vi "Get First Pt.vi"(11 "Input Traj":T1) -> (3 "First Traj Pt":dbl[](array[numeric]))   [LabVIEW 2016]
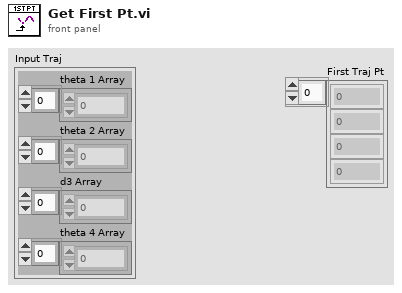
[diagram p1: front panel]
types:
  T1 = cluster{"theta 1 Array":dbl[], "theta 2 Array":dbl[], "d3 Array":dbl[], "theta 4 Array":dbl[]}
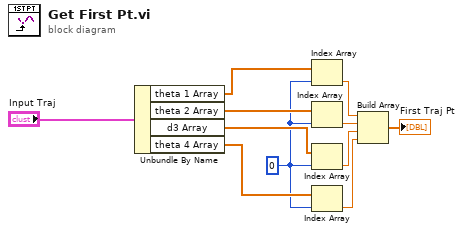
[diagram p0: block diagram]
diagram:
  w2 = 0 ("index")
  n1 = Unbundle By Name("Input Traj") -> ("theta 1 Array"=w11:dbl[], "theta 2 Array"=w5:dbl[], "d3 Array"=w4:dbl[], "theta 4 Array"=w3:dbl[])
  n2 = Index Array(array=w11, index=w2) -> (element=w10:dbl)
  n3 = Index Array(array=w5, index=w2) -> (element=w9:dbl)
  n4 = Index Array(array=w4, index=w2) -> (element=w8:dbl)
  n5 = Index Array(array=w3, index=w2) -> (element=w7:dbl)
  n6 = Build Array(w10, w9, w8, w7) -> (→"First Traj Pt":dbl[])
